vi "home.vi"   [LabVIEW 2020]
uses:
  <vilib>/Motion/Express/_s/nimc.ex.findReferenceMove.startReferenceMove.axis.modeHome.vi
  <vilib>/Motion/BlockNode/FB.NIMotion.xnode
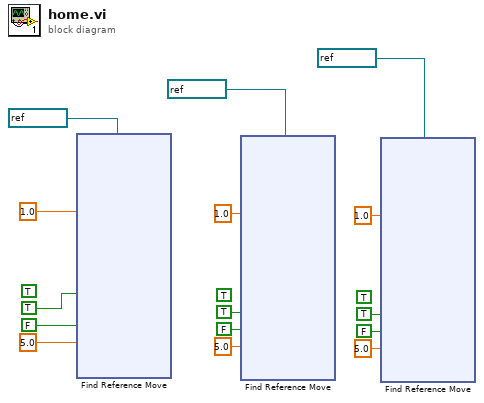
[diagram p0: block diagram]
diagram:
  (unwired) TRUE ("stop on forward edge")
  (unwired) TRUE ("stop on forward edge")
  (unwired) TRUE ("stop on forward edge")
  n1 = xnode ("Find Reference Move")("stop on forward edge"=TRUE, "approach forward"=FALSE, "approach velocity"=5.0, "resource"=refnum<k21> "Axis 3", "acceleration"=1.0) -> ()  [unwired: 8 in, 3 out]
  n2 = xnode ("Find Reference Move")("stop on forward edge"=TRUE, "approach forward"=FALSE, "approach velocity"=5.0, "resource"=refnum<k21> "Axis 1", "acceleration"=1.0) -> ()  [unwired: 8 in, 3 out]
  n3 = xnode ("Find Reference Move")("stop on forward edge"=TRUE, "approach forward"=FALSE, "approach velocity"=5.0, "resource"=refnum<k21> "Axis 2", "acceleration"=1.0) -> ()  [unwired: 8 in, 3 out]
